vi "Launch All Modules.vi"(8 "error in":errorcluster) -> (0 "error out":errorcluster)   [LabVIEW 2018]
doc: "All Rights Reserved © 2017 SyncSols"
uses:
  Controls/Main Engine Hardware Info Data Cluster.ctl
  Controls/Main Engine DAQ Device Info.ctl
  Controls/Main Engine Serial Card Details.ctl
panel:
  in  "Serial Device Info":T1[](array[typedef])
  in  "DAQ Device Info":T2[](array[typedef])
  in  "# of 429 Modules":i32
  in  "# of 1553 Modules":i32
  in  "Hardware Info":T3[](array[typedef]) {"Is Present?" items=["Initializing"=-2, "Unknown"=-1, "Not Present"=0, "Present"=1]}
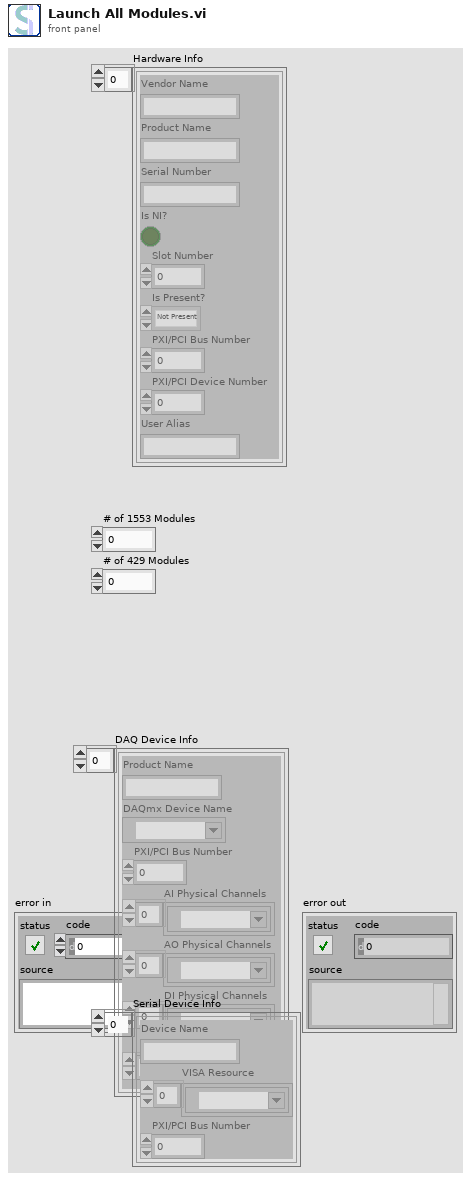
[diagram p1: front panel]
types:
  T1 = typedef "Main Engine Serial Card Details.ctl" = cluster{"Device Name":string, "VISA Resource":refnum<visa-resource-name>[], "PXI/PCI Bus Number":u32}
  T2 = typedef "Main Engine DAQ Device Info.ctl" = cluster{"Product Name":string, "DAQmx Device Name":tag, "PXI/PCI Bus Number":u32, "AI Physical Channels":tag[], "AO Physical Channels":tag[], "DI Physical Channels":tag[], "DO Physical Channel":tag[]}
  T3 = typedef "Main Engine Hardware Info Data Cluster.ctl" = cluster{"Vendor Name":string, "Product Name":string, "Serial Number":string, "Is NI?":bool, "Slot Number":i32, "Is Present?":i32, "PXI/PCI Bus Number":u32, "PXI/PCI Device Number":u32, "User Alias":string}
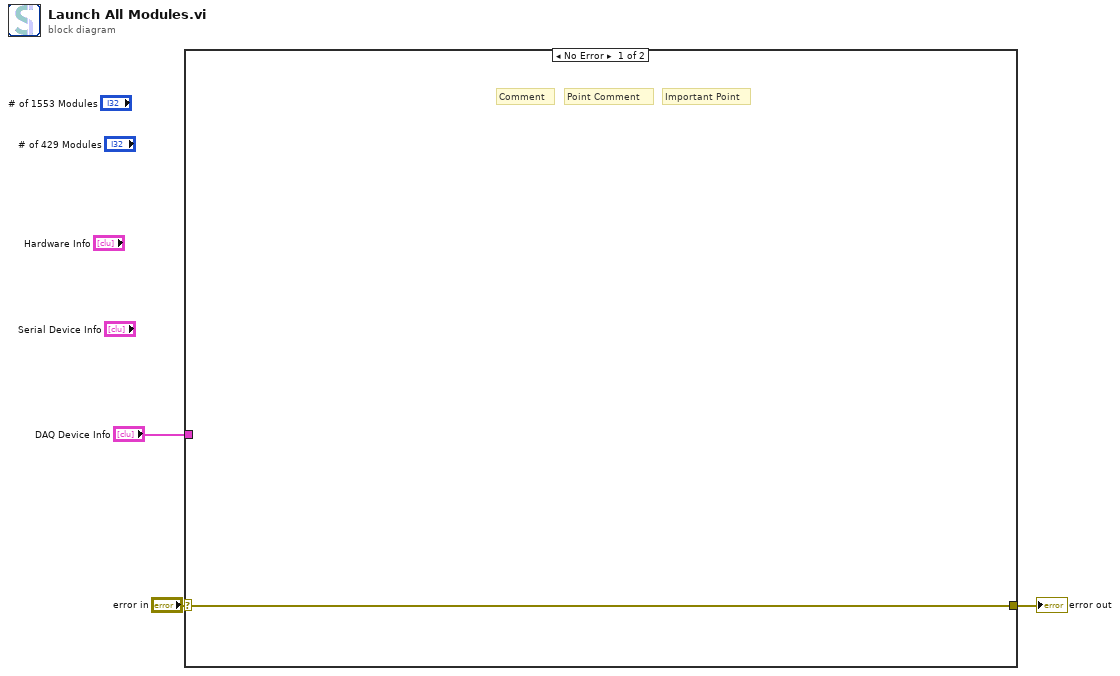
[diagram p0: block diagram]
diagram:
  n1 = case shown="No Error" "error in" {
    selector: "error in" -> [w4 w5]
    tunnel: [w4 w5] -> w3
    tunnel: "DAQ Device Info" -> [_ _]
    frame No Error {
      # "Important Point"
      # "Point Comment"
      # "Comment"
    }
    frame Error {
    }
  }
  "error out" <- w3
